vi "Find Exe Path.vi"(8 "error in (no error)":errorcluster, 10 "executable":string) -> (0 "error out":errorcluster, 2 "path":path)   [LabVIEW 2013, in "libssh2_integration_tests.lvlib" / "Server Fixture.lvclass"]
doc: "Find the path of an executable.\n\nThe executable must be registered in the PATH environment variable."
uses:
  Server Fixture.lvclass
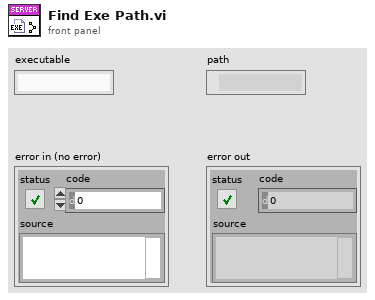
[diagram p1: front panel]
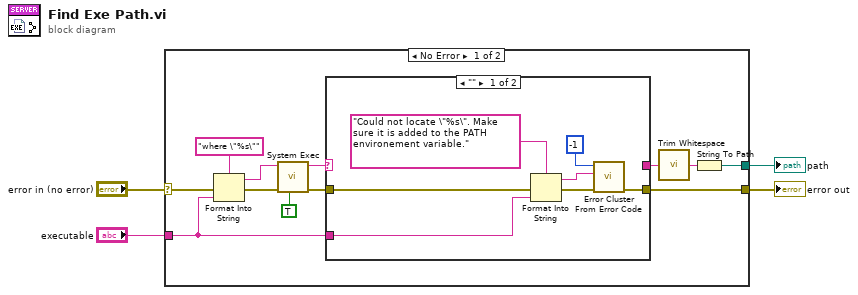
[diagram p0: block diagram]
diagram:
  n1 = case shown="No Error" "error in (no error)" {
    selector: "error in (no error)" -> [w6 w26]
    tunnel: "executable" -> [w10 _]
    tunnel: [w8 _] -> w3
    tunnel: [w7 w26] -> w2
    frame No Error {
      n2 = Format Into String(format string="where \"%s\"" ("standard input"), error in=w6, w10) -> (resulting string=w15:string, error out=w13:errorcluster)  [unwired: 1 in]
      n3 = call <vilib>:"System Exec.vi"("run minimized? (F)"=TRUE, "error in (no error)"=w13, "command line"=w15) -> ("error out"=w11:errorcluster, "standard output"=w12:string)  [unwired: 5 in, 2 out]
      n4 = case shown="\"\"" w12 {
        selector: w12 -> [_ w25]
        tunnel: [_ w25] -> w9
        tunnel: [w22 w24] -> w7
        tunnel: w11 -> [w23 w24]
        tunnel: w10 -> [w18 _]
        frame "" {
          n5 = Format Into String(format string="Could not locate \"%s\". Make sure it is added to the PATH environement variable." ("error message (\"\")"), error in=w23, w18) -> (resulting string=w17:string, error out=w21:errorcluster)  [unwired: 1 in]
          n6 = call <vilib>:"Error Cluster From Error Code.vi"("error in (no error)"=w21, "error message (\"\")"=w17, "error code (0)"=-1) -> ("error out"=w22:errorcluster)  [unwired: 6 in]
        }
        frame Default {
        }
      }
      n7 = call <vilib>:"Trim Whitespace.vi"("string"=w9) -> ("trimmed string"=w5:string)  [unwired: 1 in]
      n8 = String To Path(string=w5) -> (path=w8:path)
    }
    frame Error {
    }
  }
  "path" <- w3
  "error out" <- w2
